vi "configureCameras.vi"(8 "error in (no error)":errorcluster, 10 "deviceName":string, 11 "AtomChipHWC in":refnum<class "AtomChipHWC.lvclass">) -> (0 "error out":errorcluster, 3 "AtomChipHWC out":refnum<class "AtomChipHWC.lvclass">)   [LabVIEW 2011, in "Hardware.lvlib" / "HWControllers.lvlib" / "AtomChipHWC.lvclass"]
doc: "Configure this camera for the next acquisition"
uses:
  AtomChipHWC.lvclass
  AtomChipHWC.lvclass/AtomChipHWC.ctl
  Tools/Filing/FileSystem/FileSystem.lvclass
  IntegrationManagement/CameraManager.lvclass
  HWController.lvclass
  Tools/Filing.lvlib
  Tools/Filing/FileNeologist/FileNeologist.lvclass
  Tools/SettingsProcessors/ScriptListCompiler/ScriptListCompiler.lvclass
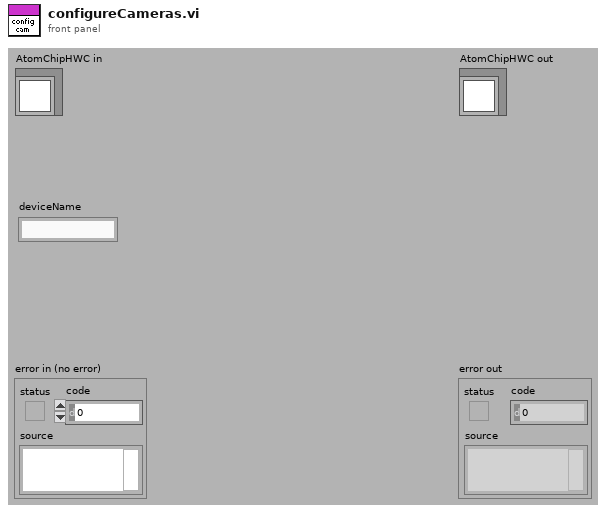
[diagram p1: front panel]
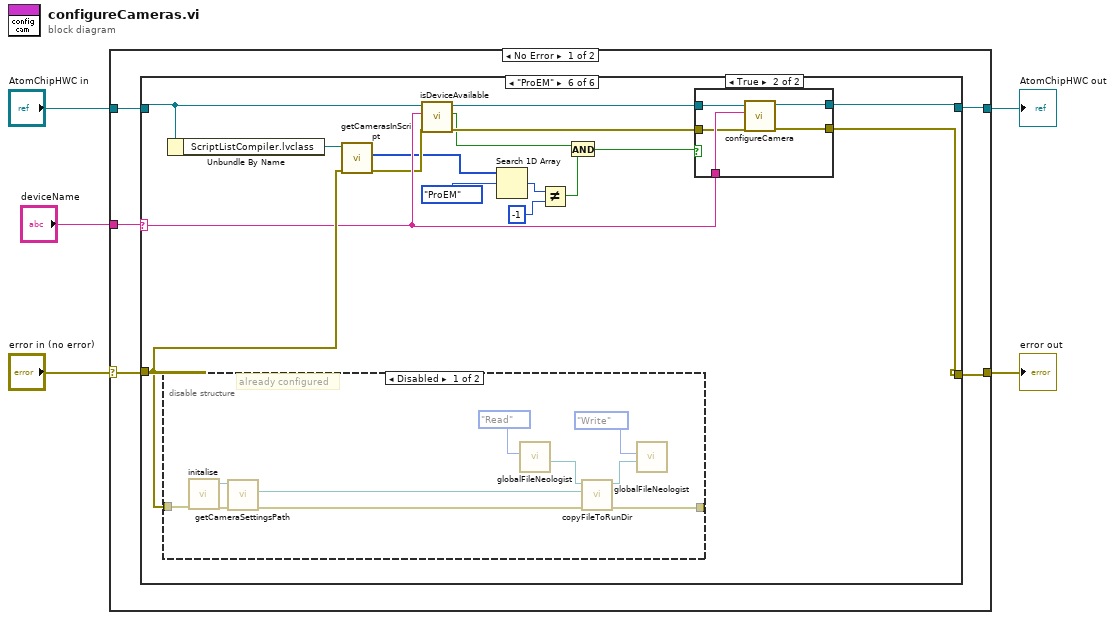
[diagram p0: block diagram]
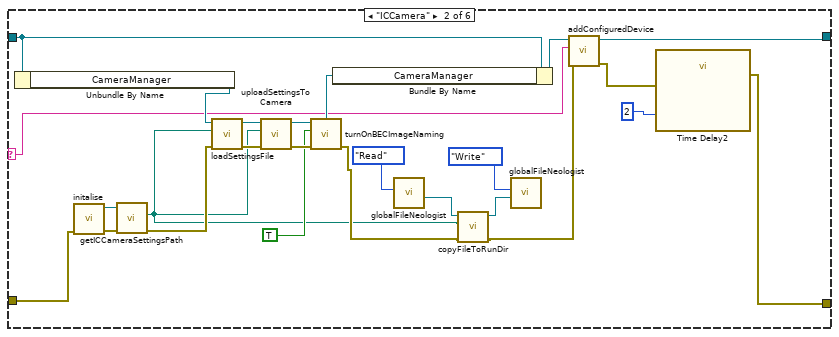
[diagram p3: hidden frame]
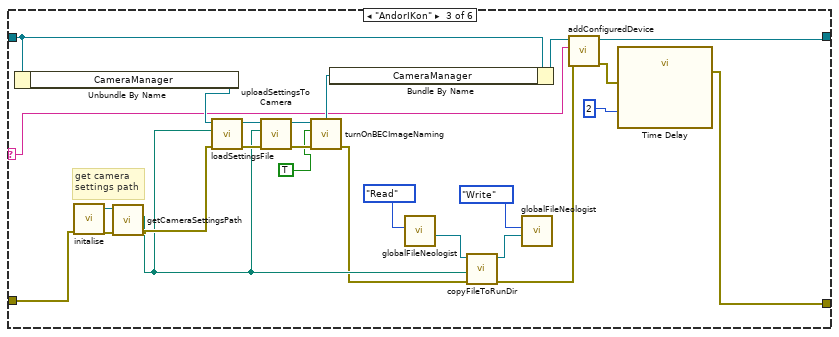
[diagram p4: hidden frame]
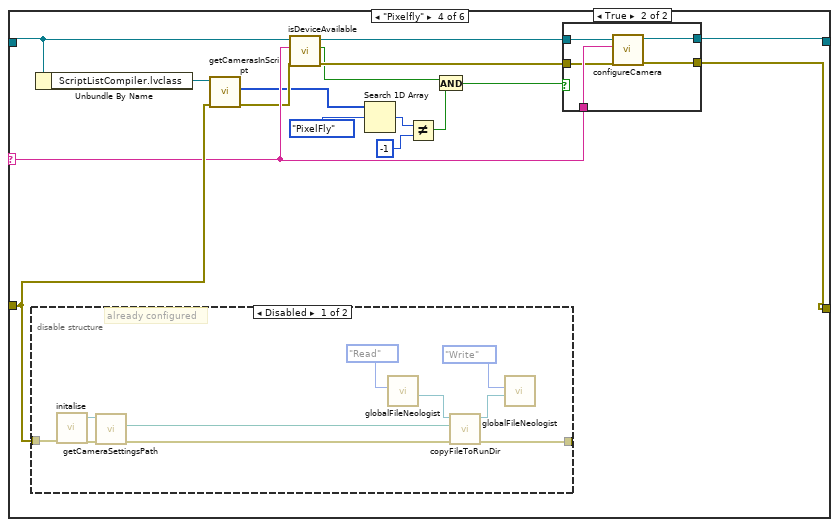
[diagram p5: hidden frame]
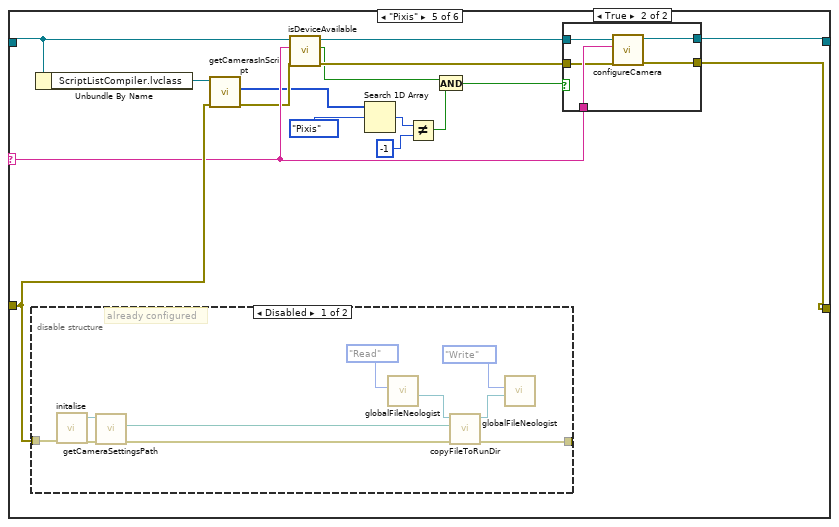
[diagram p8: hidden frame]
diagram:
  n1 = case shown="No Error" "error in (no error)" {
    selector: "error in (no error)" -> [w6 w166]
    tunnel: [w7 w166] -> w4
    tunnel: [w8 w165] -> w1
    tunnel: "AtomChipHWC in" -> [w9 w165]
    tunnel: "deviceName" -> [w10 _]
    frame No Error {
      n2 = case shown="\"ProEM\"" w10 {
        selector: w10 -> [_ w23 w51 w72 w106 w140]
        tunnel: w9 -> [w12 w37 w62 w74 w108 w142]
        tunnel: [w12 w24 w52 w77 w111 w145] -> w8
        tunnel: [w11 w13 w38 w78 w112 w146] -> w7
        tunnel: w6 -> [w11 w31 w59 w75 w109 w143]
        frame "No Hardware", Default {
        }
        frame "ICCamera" {
          n3 = Unbundle By Name(w37) -> ("CameraManager"=w34:refnum<class "CameraManager.lvclass">)
          n4 = call "initalise.vi"("error in (no error)"=w31) -> ("error out"=w36:errorcluster, "FileSystem out"=w35:refnum<class "FileSystem.lvclass">)  [unwired: 9 in]
          n5 = call-dynamic "getICCameraSettingsPath.vi"("error in (no error)"=w36, "FileSystem.lvclass in"=w35) -> ("error out"=w32:errorcluster, "ICCameraSettingsPath"=w18:path)  [unwired: 7 in, 1 out]
          n6 = call "loadSettingsFile.vi"("error in (no error)"=w32, "Path"=w18, "CameraManager in"=w34) -> ("error out"=w33:errorcluster, "CameraManager out"=w30:refnum<class "CameraManager.lvclass">)  [unwired: 7 in]
          n7 = call "uploadSettingsToCamera.vi"("error in (no error)"=w33, "Path"=w18, "CameraManager in"=w30) -> ("error out"=w28:errorcluster, "CameraManager out"=w29:refnum<class "CameraManager.lvclass">)  [unwired: 7 in]
          n8 = call "turnOnBECImageNaming.vi"("error in (no error)"=w28, "ImageRenaming"=TRUE, "CameraManager in"=w29) -> ("error out"=w20:errorcluster, "CameraManager out"=w27:refnum<class "CameraManager.lvclass">)  [unwired: 7 in]
          n9 = Bundle By Name(cluster=w37, "CameraManager"=w27) -> (w25:refnum<class "AtomChipHWC.lvclass">)
          n10 = call "globalFileNeologist.vi"("Action"=enum16{"Write", "Read"}."Read") -> ("FileNeologist out"=w17:refnum<class "FileNeologist.lvclass">)  [unwired: 10 in]
          n11 = call "copyFileToRunDir.vi"("error in (no error)"=w20, "Path"=w18, "FileNeologist in"=w17) -> ("error out"=w19:errorcluster, "FileNeologist out"=w16:refnum<class "FileNeologist.lvclass">)  [unwired: 7 in]
          n12 = call "globalFileNeologist.vi"("FileNeologist in"=w16, "Action"=enum16{"Write", "Read"}."Write") -> ()  [unwired: 9 in, 1 out]
          n13 = call "addConfiguredDevice.vi"("error in (no error)"=w19, "deviceName"=w23, "HWController in"=w25) -> ("error out"=w14:errorcluster, "HWController out"=w24:refnum<class "AtomChipHWC.lvclass">)  [unwired: 7 in]
          n14 = call "Time Delay2"("error in (no error)"=w14, "Delay Time (s)"=2) -> ("error out"=w13:errorcluster)  [unwired: 9 in]
        }
        frame "AndorIKon" {
          # "get camera\nsettings path"
          n15 = Unbundle By Name(w62) -> ("CameraManager"=w61:refnum<class "CameraManager.lvclass">)
          n16 = call "initalise.vi"("error in (no error)"=w59) -> ("error out"=w50:errorcluster, "FileSystem out"=w49:refnum<class "FileSystem.lvclass">)  [unwired: 9 in]
          n17 = call-dynamic "getCameraSettingsPath.vi"("error in (no error)"=w50, "FileSystem.lvclass in"=w49) -> ("error out"=w48:errorcluster, "CameraSettingsPath"=w47:path)  [unwired: 7 in, 1 out]
          n18 = call "loadSettingsFile.vi"("error in (no error)"=w48, "Path"=w47, "CameraManager in"=w61) -> ("error out"=w60:errorcluster, "CameraManager out"=w58:refnum<class "CameraManager.lvclass">)  [unwired: 7 in]
          n19 = call "uploadSettingsToCamera.vi"("error in (no error)"=w60, "Path"=w47, "CameraManager in"=w58) -> ("error out"=w56:errorcluster, "CameraManager out"=w57:refnum<class "CameraManager.lvclass">)  [unwired: 7 in]
          n20 = call "turnOnBECImageNaming.vi"("error in (no error)"=w56, "ImageRenaming"=TRUE, "CameraManager in"=w57) -> ("error out"=w40:errorcluster, "CameraManager out"=w55:refnum<class "CameraManager.lvclass">)  [unwired: 7 in]
          n21 = Bundle By Name(cluster=w62, "CameraManager"=w55) -> (w53:refnum<class "AtomChipHWC.lvclass">)
          n22 = call "globalFileNeologist.vi"("Action"=enum16{"Write", "Read"}."Read") -> ("FileNeologist out"=w42:refnum<class "FileNeologist.lvclass">)  [unwired: 10 in]
          n23 = call "copyFileToRunDir.vi"("error in (no error)"=w40, "Path"=w47, "FileNeologist in"=w42) -> ("error out"=w39:errorcluster, "FileNeologist out"=w41:refnum<class "FileNeologist.lvclass">)  [unwired: 7 in]
          n24 = call "globalFileNeologist.vi"("FileNeologist in"=w41, "Action"=enum16{"Write", "Read"}."Write") -> ()  [unwired: 9 in, 1 out]
          n25 = call "addConfiguredDevice.vi"("error in (no error)"=w39, "deviceName"=w51, "HWController in"=w53) -> ("error out"=w46:errorcluster, "HWController out"=w52:refnum<class "AtomChipHWC.lvclass">)  [unwired: 7 in]
          n26 = call "Time Delay"("error in (no error)"=w46, "Delay Time (s)"=2) -> ("error out"=w38:errorcluster)  [unwired: 9 in]
        }
        frame "Pixelfly" {
          n27 = disable-structure shown="Disabled" {
            disable-tunnel: w75 -> [w89 w96]
            disable-tunnel: [w86 w96] -> _
            frame Disabled {
              # "already configured"
              n28 = call "initalise.vi"("error in (no error)"=w89) -> ("error out"=w91:errorcluster, "FileSystem out"=w90:refnum<class "FileSystem.lvclass">)  [unwired: 9 in]
              n29 = call-dynamic "getCameraSettingsPath.vi"("error in (no error)"=w91, "FileSystem.lvclass in"=w90) -> ("error out"=w87:errorcluster, "CameraSettingsPath"=w88:path)  [unwired: 7 in, 1 out]
              n30 = call "globalFileNeologist.vi"("Action"=enum16{"Write", "Read"}."Read") -> ("FileNeologist out"=w93:refnum<class "FileNeologist.lvclass">)  [unwired: 10 in]
              n31 = call "copyFileToRunDir.vi"("error in (no error)"=w87, "Path"=w88, "FileNeologist in"=w93) -> ("error out"=w86:errorcluster, "FileNeologist out"=w92:refnum<class "FileNeologist.lvclass">)  [unwired: 7 in]
              n32 = call "globalFileNeologist.vi"("FileNeologist in"=w92, "Action"=enum16{"Write", "Read"}."Write") -> ()  [unwired: 9 in, 1 out]
            }
            frame Enabled {
            }
          }
          n33 = Unbundle By Name(w74) -> ("ScriptListCompiler.lvclass"=w76:refnum<class "ScriptListCompiler.lvclass">)
          n34 = call "getCamerasInScript.vi"("error in (no error)"=w75, "ScriptListCompiler in"=w76) -> ("error out"=w71:errorcluster, "camerasInScript"=w69:enum16{"Pixis", "ProEM", "PixelFly"}[])  [unwired: 7 in, 1 out]
          n35 = call "isDeviceAvailable.vi"("error in (no error)"=w71, "device"=w72, "HWController in"=w74) -> ("error out"=w70:errorcluster, "available"=w64:bool, "HWController out"=w73:refnum<class "AtomChipHWC.lvclass">)  [unwired: 6 in]
          n36 = Search 1D Array(1D array=w69, element=enum16{"Pixis", "ProEM", "PixelFly"}."PixelFly" ("Camera")) -> (index of element=w67:i32)  [unwired: 1 in]
          n37 = Not Equal?(x=w67, y=-1) -> (x != y?=w65:bool)
          n38 = And(x=w64, y=w65) -> (x .and. y?=w63:bool)
          n39 = case shown="True" w63 {
            tunnel: [w79 w85] -> w78
            tunnel: [w80 w84] -> w77
            tunnel: w73 -> [w80 w83]
            tunnel: w72 -> [_ w82]
            tunnel: w70 -> [w79 w81]
            frame False {
            }
            frame True {
              n40 = call "configureCamera.vi"("error in (no error)"=w81, "device"=w82, "AtomChipHWC in"=w83) -> ("error out"=w85:errorcluster, "AtomChipHWC out"=w84:refnum<class "AtomChipHWC.lvclass">)  [unwired: 7 in]
            }
          }
        }
        frame "Pixis" {
          n41 = disable-structure shown="Disabled" {
            disable-tunnel: w109 -> [w123 w130]
            disable-tunnel: [w120 w130] -> _
            frame Disabled {
              # "already configured"
              n42 = call "initalise.vi"("error in (no error)"=w123) -> ("error out"=w125:errorcluster, "FileSystem out"=w124:refnum<class "FileSystem.lvclass">)  [unwired: 9 in]
              n43 = call-dynamic "getCameraSettingsPath.vi"("error in (no error)"=w125, "FileSystem.lvclass in"=w124) -> ("error out"=w121:errorcluster, "CameraSettingsPath"=w122:path)  [unwired: 7 in, 1 out]
              n44 = call "globalFileNeologist.vi"("Action"=enum16{"Write", "Read"}."Read") -> ("FileNeologist out"=w127:refnum<class "FileNeologist.lvclass">)  [unwired: 10 in]
              n45 = call "copyFileToRunDir.vi"("error in (no error)"=w121, "Path"=w122, "FileNeologist in"=w127) -> ("error out"=w120:errorcluster, "FileNeologist out"=w126:refnum<class "FileNeologist.lvclass">)  [unwired: 7 in]
              n46 = call "globalFileNeologist.vi"("FileNeologist in"=w126, "Action"=enum16{"Write", "Read"}."Write") -> ()  [unwired: 9 in, 1 out]
            }
            frame Enabled {
            }
          }
          n47 = Unbundle By Name(w108) -> ("ScriptListCompiler.lvclass"=w110:refnum<class "ScriptListCompiler.lvclass">)
          n48 = call "getCamerasInScript.vi"("error in (no error)"=w109, "ScriptListCompiler in"=w110) -> ("error out"=w105:errorcluster, "camerasInScript"=w103:enum16{"Pixis", "ProEM", "PixelFly"}[])  [unwired: 7 in, 1 out]
          n49 = call "isDeviceAvailable.vi"("error in (no error)"=w105, "device"=w106, "HWController in"=w108) -> ("error out"=w104:errorcluster, "available"=w98:bool, "HWController out"=w107:refnum<class "AtomChipHWC.lvclass">)  [unwired: 6 in]
          n50 = Search 1D Array(1D array=w103, element=enum16{"Pixis", "ProEM", "PixelFly"}."Pixis" ("Camera")) -> (index of element=w101:i32)  [unwired: 1 in]
          n51 = Not Equal?(x=w101, y=-1) -> (x != y?=w99:bool)
          n52 = And(x=w98, y=w99) -> (x .and. y?=w97:bool)
          n53 = case shown="True" w97 {
            tunnel: [w113 w119] -> w112
            tunnel: [w114 w118] -> w111
            tunnel: w107 -> [w114 w117]
            tunnel: w106 -> [_ w116]
            tunnel: w104 -> [w113 w115]
            frame False {
            }
            frame True {
              n54 = call "configureCamera.vi"("error in (no error)"=w115, "device"=w116, "AtomChipHWC in"=w117) -> ("error out"=w119:errorcluster, "AtomChipHWC out"=w118:refnum<class "AtomChipHWC.lvclass">)  [unwired: 7 in]
            }
          }
        }
        frame "ProEM" {
          n55 = disable-structure shown="Disabled" {
            disable-tunnel: w143 -> [w157 w164]
            disable-tunnel: [w154 w164] -> _
            frame Disabled {
              # "already configured"
              n56 = call "initalise.vi"("error in (no error)"=w157) -> ("error out"=w159:errorcluster, "FileSystem out"=w158:refnum<class "FileSystem.lvclass">)  [unwired: 9 in]
              n57 = call-dynamic "getCameraSettingsPath.vi"("error in (no error)"=w159, "FileSystem.lvclass in"=w158) -> ("error out"=w155:errorcluster, "CameraSettingsPath"=w156:path)  [unwired: 7 in, 1 out]
              n58 = call "globalFileNeologist.vi"("Action"=enum16{"Write", "Read"}."Read") -> ("FileNeologist out"=w161:refnum<class "FileNeologist.lvclass">)  [unwired: 10 in]
              n59 = call "copyFileToRunDir.vi"("error in (no error)"=w155, "Path"=w156, "FileNeologist in"=w161) -> ("error out"=w154:errorcluster, "FileNeologist out"=w160:refnum<class "FileNeologist.lvclass">)  [unwired: 7 in]
              n60 = call "globalFileNeologist.vi"("FileNeologist in"=w160, "Action"=enum16{"Write", "Read"}."Write") -> ()  [unwired: 9 in, 1 out]
            }
            frame Enabled {
            }
          }
          n61 = Unbundle By Name(w142) -> ("ScriptListCompiler.lvclass"=w144:refnum<class "ScriptListCompiler.lvclass">)
          n62 = call "getCamerasInScript.vi"("error in (no error)"=w143, "ScriptListCompiler in"=w144) -> ("error out"=w139:errorcluster, "camerasInScript"=w137:enum16{"Pixis", "ProEM", "PixelFly"}[])  [unwired: 7 in, 1 out]
          n63 = call "isDeviceAvailable.vi"("error in (no error)"=w139, "device"=w140, "HWController in"=w142) -> ("error out"=w138:errorcluster, "available"=w132:bool, "HWController out"=w141:refnum<class "AtomChipHWC.lvclass">)  [unwired: 6 in]
          n64 = Search 1D Array(1D array=w137, element=enum16{"Pixis", "ProEM", "PixelFly"}."ProEM" ("Camera")) -> (index of element=w135:i32)  [unwired: 1 in]
          n65 = Not Equal?(x=w135, y=-1) -> (x != y?=w133:bool)
          n66 = And(x=w132, y=w133) -> (x .and. y?=w131:bool)
          n67 = case shown="True" w131 {
            tunnel: [w147 w153] -> w146
            tunnel: [w148 w152] -> w145
            tunnel: w141 -> [w148 w151]
            tunnel: w140 -> [_ w150]
            tunnel: w138 -> [w147 w149]
            frame False {
            }
            frame True {
              n68 = call "configureCamera.vi"("error in (no error)"=w149, "device"=w150, "AtomChipHWC in"=w151) -> ("error out"=w153:errorcluster, "AtomChipHWC out"=w152:refnum<class "AtomChipHWC.lvclass">)  [unwired: 7 in]
            }
          }
        }
      }
    }
    frame Error {
    }
  }
  "error out" <- w4
  "AtomChipHWC out" <- w1
